vi "AlliGator Check Missing Python Plugin Doc String.vi"(8 "error in (no error)":errorcluster, 9 "Source":string, 11 "Doc String Found":bool) -> (0 "error out":errorcluster)   [LabVIEW 2021, in "AlliGator Python Plugins.lvlib"]
doc: "Outputs warning with missing doc string message."
uses:
  <vilib>/Utility/error.llb/DialogType.ctl
  AlliGator Python Plugins.lvlib
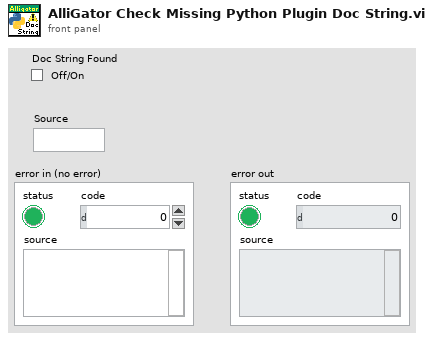
[diagram p1: front panel]
types:
  T1 = typedef "DialogType.ctl" = u16
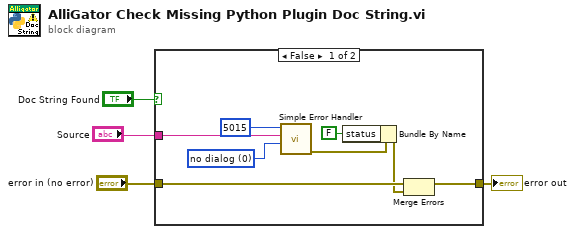
[diagram p0: block diagram]
diagram:
  n1 = case shown="False" "Doc String Found" {
    tunnel: [w8 w13] -> w4
    tunnel: "error in (no error)" -> [w7 w13]
    tunnel: "Source" -> [w10 _]
    frame False {
      w9 = T1 0 items=["no dialog", "OK message", "continue or stop message", "OK message + warnings", "continue/stop + warnings"] ("type of dialog (OK msg:1)")
      n2 = call <vilib>:"Simple Error Handler.vi"("error code (no error:0)"=5015, "error source (\" \")"=w10, "type of dialog (OK msg:1)"=w9) -> ("error out"=w12:errorcluster)  [unwired: 2 in, 4 out]
      n3 = Bundle By Name(cluster=w12, "status"=FALSE) -> (w6:errorcluster)
      n4 = Merge Errors(w7, w6) -> (w8:errorcluster)
    }
    frame True {
    }
  }
  "error out" <- w4
